vi "Append Watermark Image.vi"(0 "PDF Report IN":refnum<class "PDF Report Class.lvclass">, 2 "Watermark Image":T1={"Image path"=path "", "Opacity (%)"=10.0, "Postion"={"Position"=enum."Center (text section)", "X"=0.0, "Y"=0.0}, "Automatic"=FALSE, "Scale(%)"=100.0, "Rotate(°)"=0.0}, 11 "error in (no error)":errorcluster) -> (4 "PDF Report OUT":refnum<class "PDF Report Class.lvclass">, 15 "error out":errorcluster)   [LabVIEW 2019]
doc: "Appends a <B>watermark</B> (text or image) on each page of the PDF report. \n\n<B>FRANÇAIS</B>\nAjoute un <B>filigrane</B> (texte or image) sur chaque page du rapport PDF. \n\nVersion 1.0\nDeveloped by Jean-Marc Simard\nCopyright © 2010, Exaprom Inc.\nAll rights reserved.\nLicense: BSD\n\nWith iTextSharp Library\n(http://itextsharp.sourceforge.net)"
uses:
  <userlib>/Exaprom PDF/LV Class/PDF Report Class/PDF Report Class.lvclass
  <userlib>/Exaprom PDF/Controls/Header, Footer and Watermark Controls/Watermark Image Cluster.ctl
  <userlib>/Exaprom PDF/Controls/Header, Footer and Watermark Controls/Watermark Position.ctl
  <userlib>/Exaprom PDF/Controls/Header, Footer and Watermark Controls/Header footer horiz alignment.ctl
  <userlib>/Exaprom PDF/Controls/Font Controls/Font complete cluster.ctl
  <userlib>/Exaprom PDF/Controls/Font Controls/Font size.ctl
  <userlib>/Exaprom PDF/Controls/Font Controls/Font color.ctl
  <userlib>/Exaprom PDF/Controls/Font Controls/Type and encoding.ctl
  <userlib>/Exaprom PDF/Controls/Text Controls/Unicode/Type and run direction.ctl
  C:/Program Files/National Instruments/LabVIEW 2019/user.lib/Exaprom PDF/DLL/itextsharp.dll
  DLL/itextsharp.dll
  <userlib>/Exaprom PDF/LV Class/Fonts Class/Font Class.lvclass
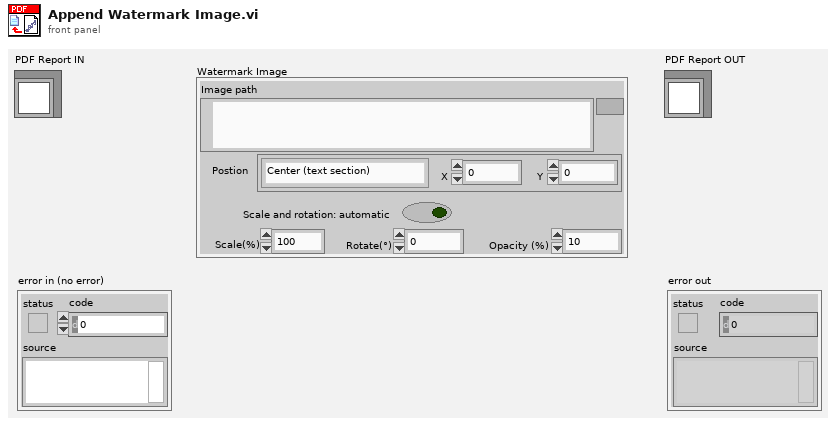
[diagram p1: front panel]
types:
  T1 = typedef "Watermark Image Cluster.ctl" = cluster{"Image path":path, "Opacity (%)":sgl, "Postion":cluster{"Position":T2, "X":sgl, "Y":sgl}, "Automatic":bool, "Scale(%)":sgl, "Rotate(°)":sgl}
  T2 = typedef "Watermark Position.ctl" = enum16{"Absolute", "Center (page)", "Center (text section)"}
  T3 = typedef "Header footer horiz alignment.ctl" = enum16{"Left", "Center", "Right"}
  T4 = typedef "Font complete cluster.ctl" = cluster{"Name":string, "Size":T5, "Color":T6, "Style":cluster{"Bold":bool, "Italic":bool, "Underline":bool, "Strikeout":bool}, "Type":T7}
  T5 = typedef "Font size.ctl" = sgl
  T6 = typedef "Font color.ctl" = u32
  T7 = typedef "Type and encoding.ctl" = cluster{"Type&direction":T8, "Embedded":bool, "Encoding":string}
  T8 = typedef "Type and run direction.ctl" = enum16{"Select", "ASCII", "UTF-16", "UTF-16 (default)", "UTF-16 (LTR)", "UTF-16 (RTL)"}
  T9 = typedef "Watermark cluster2.ctl" = cluster{"Show? (F)":bool, "Type":enum16{"Image", "Text"}, "Opacity (%)":sgl, "Rotate(°)":sgl, "Position":cluster{"Position":T2, "X":sgl, "Y":sgl}, "Image path":path, "Scaled(%)":sgl, "Image refnum":refnum<k24>, "Text":string, "Font":cluster{"Name":string, "Size":T5, "Color":T6}, "Font refnum":refnum<k24>, "Alignment":T3, "Automatic":bool}
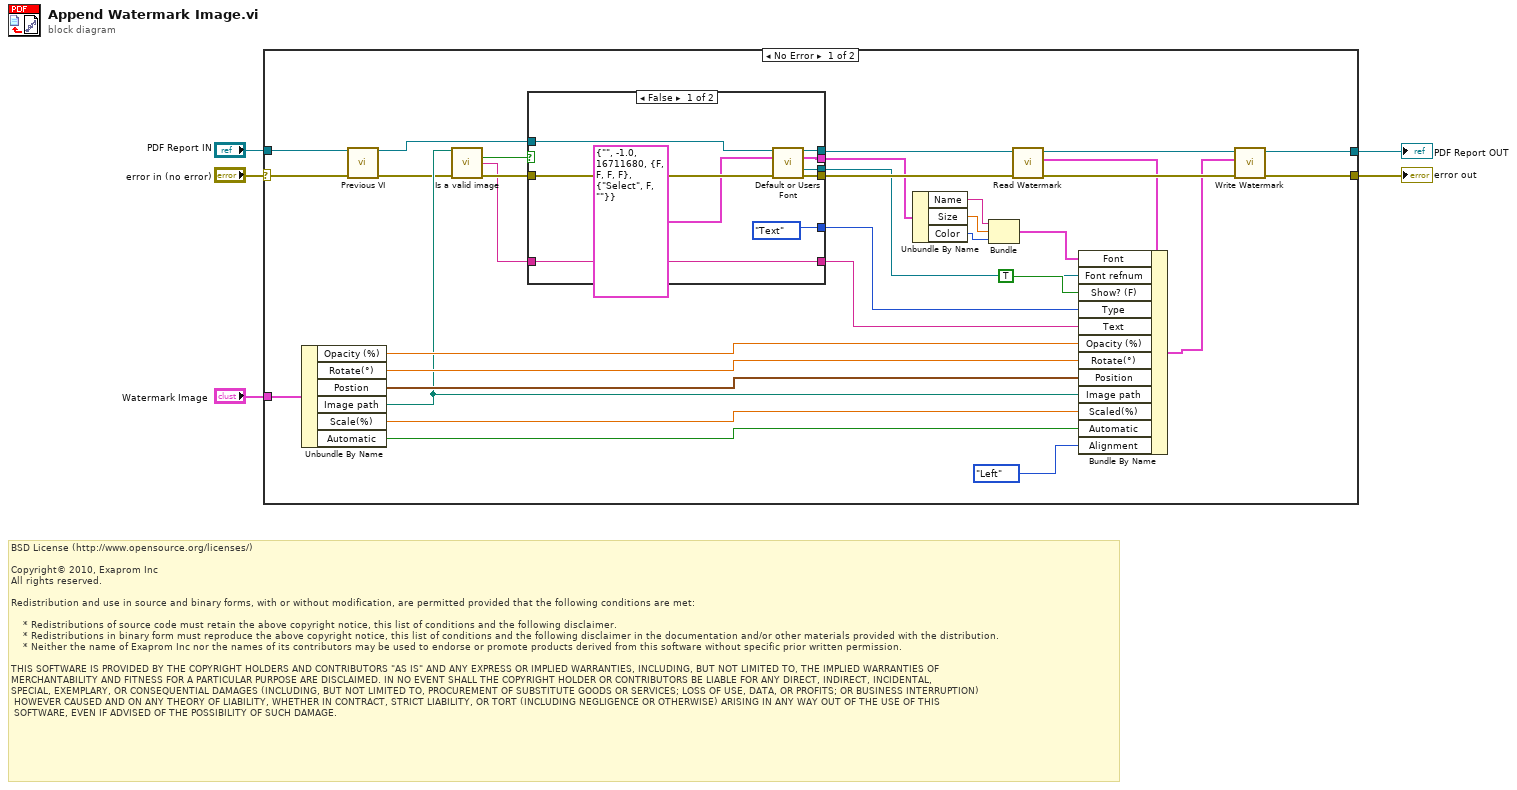
[diagram p0: block diagram]
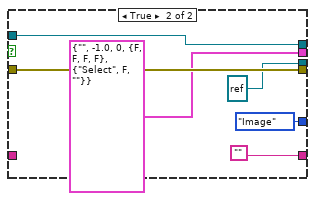
[diagram p2: hidden frame]
diagram:
  # "BSD License (http://www.opensource.org/licenses/)\n\nCopyright© 2010, Exaprom Inc\nAll rights reserved.\n\nRedistribution and use in source and binary forms, with or without modification, are permitted provided that the following conditions are met:\n\n    * Redistributions of source code must retain the above copyright notice, this list of conditions and the following disclaimer.\n    * Redistributions in binary form must reproduce the above copyright notice, this list of conditions and the following disclaimer in the documentation and/or other materials provided with the distribution.\n    * Neither the name of Exaprom Inc nor the names of its contributors may be used to endorse or promote products derived from this software without specific prior written permission.\n\nTHIS SOFTWARE IS PROVIDED BY THE COPYRIGHT HOLDERS AND CONTRIBUTORS \"AS IS\" AND ANY EXPRESS OR IMPLIED WARRANTIES, INCLUDING, BUT NOT LIMITED TO, THE IMPLIED WARRANTIES OF \nMERCHANTABILITY AND FITNESS FOR A PARTICULAR PURPOSE ARE DISCLAIMED. IN NO EVENT SHALL THE COPYRIGHT HOLDER OR CONTRIBUTORS BE LIABLE FOR ANY DIRECT, INDIRECT, INCIDENTAL,\nSPECIAL, EXEMPLARY, OR CONSEQUENTIAL DAMAGES (INCLUDING, BUT NOT LIMITED TO, PROCUREMENT OF SUBSTITUTE GOODS OR SERVICES; LOSS OF USE, DATA, OR PROFITS; OR BUSINESS INTERRUPTION)\n HOWEVER CAUSED AND ON ANY THEORY OF LIABILITY, WHETHER IN CONTRACT, STRICT LIABILITY, OR TORT (INCLUDING NEGLIGENCE OR OTHERWISE) ARISING IN ANY WAY OUT OF THE USE OF THIS\n SOFTWARE, EVEN IF ADVISED OF THE POSSIBILITY OF SUCH DAMAGE."
  n1 = case shown="No Error" "error in (no error)" {
    selector: "error in (no error)" -> [w36 w54]
    tunnel: "PDF Report IN" -> [w37 w53]
    tunnel: "Watermark Image" -> [w35 _]
    tunnel: [w6 w53] -> w3
    tunnel: [w9 w54] -> w2
    frame No Error {
      n2 = Unbundle By Name(w35) -> ("Opacity (%)"=w34:sgl, "Rotate(°)"=w33:sgl, "Postion"=w32:cluster{"Position":T2, "X":sgl, "Y":sgl}, "Image path"=w24:path, "Scale(%)"=w31:sgl, "Automatic"=w29:bool)
      n3 = call <userlib>:"Previous VI.vi"("PDF Report IN"=w37, "error in (no error)"=w36) -> ("PDF Report OUT"=w23:refnum<class "PDF Report Class.lvclass">, "error out"=w22:errorcluster)  [unwired: 12 out]
      n4 = call <userlib>:"Is a valid image.vi"("Image path"=w24, "error in (no error)"=w22) -> ("Valid Image?"=w25:bool, "Message"=w26:string, "error out"=w27:errorcluster)  [unwired: 11 out]
      n5 = case shown="False" w25 {
        tunnel: [enum16{"Image", "Text"}."Text" ("Watermark .Type") enum16{"Image", "Text"}."Image" ("Watermark .Type")] -> w15
        tunnel: [w46 ""] -> w14
        tunnel: w26 -> [w46 _]
        tunnel: [w44 w52] -> w10
        tunnel: w23 -> [w45 w52]
        tunnel: w27 -> [w43 w51]
        tunnel: [w42 T4 {"Name"="", "Size"=-1.0, "Color"=0, "Style"={"Bold"=FALSE, "Italic"=FALSE, "Underline"=FALSE, "Strikeout"=FALSE}, "Type"={"Type&direction"=enum."Select", "Embedded"=FALSE, "Encoding"=""}} ("Font OUT")] -> w20
        tunnel: [w41 refnum<k24> refnum ("Font Ref")] -> w16
        tunnel: [w40 w51] -> w21
        frame False {
          n6 = call <userlib>:"Default or Users Font.vi"("PDF Report"=w45, "Font"=T4 {"Name"="", "Size"=-1.0, "Color"=16711680, "Style"={"Bold"=FALSE, "Italic"=FALSE, "Underline"=FALSE, "Strikeout"=FALSE}, "Type"={"Type&direction"=enum."Select", "Embedded"=FALSE, "Encoding"=""}} ("Font OUT"), "error in (no error)"=w43) -> ("PDF Report duplicate"=w44:refnum<class "PDF Report Class.lvclass">, "Font OUT"=w42:T4, "Font Ref"=w41:refnum<k24>, "error out"=w40:errorcluster)  [unwired: 7 in, 2 out]
        }
        frame True {
        }
      }
      n7 = Unbundle By Name(w20) -> ("Name"=w19:string, "Size"=w18:T5, "Color"=w17:T6)
      n8 = Bundle("Name"=w19, "Size"=w18, "Color"=w17) -> (w28:cluster{"Name":string, "Size":T5, "Color":T6})  [unwired: 1 out]
      n9 = call-dynamic "Read Watermark .vi"("error in (no error)"=w21, "PDF Report Class in"=w10) -> ("error out"=w12:errorcluster, "Watermark Cluster"=w11:T9, "PDF Report Class out"=w7:refnum<class "PDF Report Class.lvclass">)  [unwired: 7 in]
      n10 = Bundle By Name(cluster=w11, "Font"=w28, "Font refnum"=w16, "Show? (F)"=TRUE ("Watermark .Show? (F)"), "Type"=w15, "Text"=w14, "Opacity (%)"=w34, "Rotate(°)"=w33, "Position"=w32, "Image path"=w24, "Scaled(%)"=w31, "Automatic"=w29, "Alignment"=Header_footer_horiz_alignment."Left" ("Watermark .Alignment")) -> (w8:T9)
      n11 = call-dynamic "Write Watermark .vi"("error in (no error)"=w12, "Watermark Cluster"=w8, "PDF Report Class in"=w7) -> ("error out"=w9:errorcluster, "PDF Report Class out"=w6:refnum<class "PDF Report Class.lvclass">)  [unwired: 7 in]
    }
    frame Error {
    }
  }
  "PDF Report OUT" <- w3
  "error out" <- w2
